vi "Configure Analog Gen Arbitrary Waveform.vi"(4 "Column Select (0)":i32, 5 "Enable Waveform (T: Enable)":bool=TRUE, 6 "Output Rate (10 %)":dbl=10.0, 7 "Load File (\"MyFile.arb\")":string="\"MyFile.arb\"", 8 "error in (no error)":errorcluster, 9 "Amplitude (0 Vrms)":dbl, 10 "Channel (0: A)":i32(ring) items=["A", "B"], 11 "VISA resource name":refnum<visa-resource-name>) -> (0 "error out":errorcluster, 3 "VISA resource name out":refnum<visa-resource-name>)   [LabVIEW 2014, in "Stanford Research SR1.lvlib"]
doc: "Configures the attributes of the Analog Generator Arbitrary Waveform."
uses:
  Stanford Research SR1.lvlib
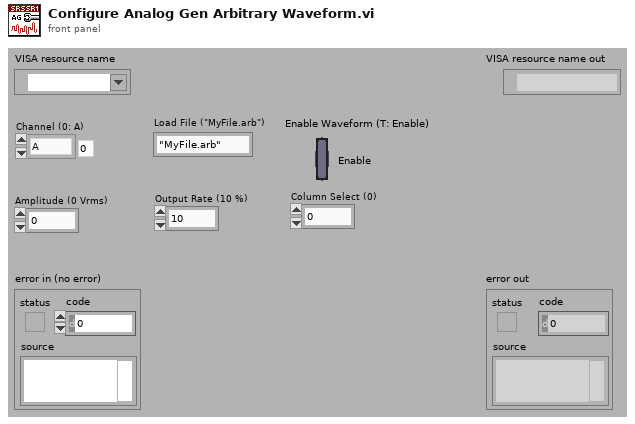
[diagram p1: front panel]
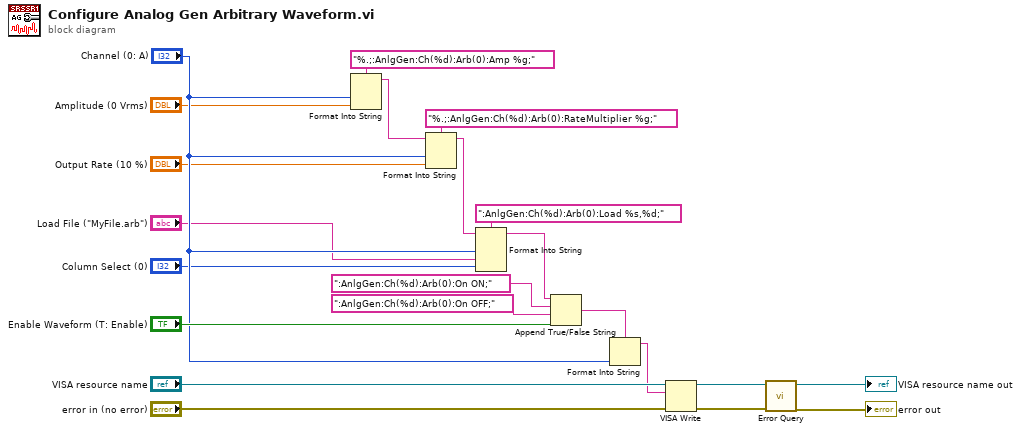
[diagram p0: block diagram]
diagram:
  n1 = Format Into String(format string="%.;:AnlgGen:Ch(%d):Arb(0):Amp %g;", "Channel (0: A)", "Amplitude (0 Vrms)") -> (resulting string=w21:string)  [unwired: 2 in, 1 out]
  n2 = Format Into String(format string="%.;:AnlgGen:Ch(%d):Arb(0):RateMultiplier %g;", initial string=w21, "Channel (0: A)", "Output Rate (10 %)") -> (resulting string=w19:string)  [unwired: 1 in, 1 out]
  n3 = Format Into String(format string=":AnlgGen:Ch(%d):Arb(0):Load %s,%d;", initial string=w19, "Channel (0: A)", "Load File (\"MyFile.arb\")", "Column Select (0)") -> (resulting string=w17:string)  [unwired: 1 in, 1 out]
  n4 = Append True/False String(1:"Enable Waveform (T: Enable)", 2:":AnlgGen:Ch(%d):Arb(0):On OFF;", 3:":AnlgGen:Ch(%d):Arb(0):On ON;", 4:w17) -> (0:w7:string)
  n5 = Format Into String(format string=w7, "Channel (0: A)") -> (resulting string=w6:string)  [unwired: 2 in, 1 out]
  n6 = VISA Write(VISA resource name="VISA resource name", write buffer=w6, error in (no error)="error in (no error)") -> (VISA resource name out=w11:refnum<visa-resource-name>, error out=w10:errorcluster)  [unwired: 1 out]
  n7 = call "Error Query.vi"("error in (no error)"=w10, "VISA resource name"=w11) -> ("error out"=→"error out":errorcluster, "VISA resource name out"=→"VISA resource name out":refnum<visa-resource-name>)  [unwired: 6 in, 2 out]
